vi "2.4b.vi"() -> ()   [LabVIEW 2020]
panel:
  out "output array 2":string[](array[string])
  in  "Array":string[][](array[string])
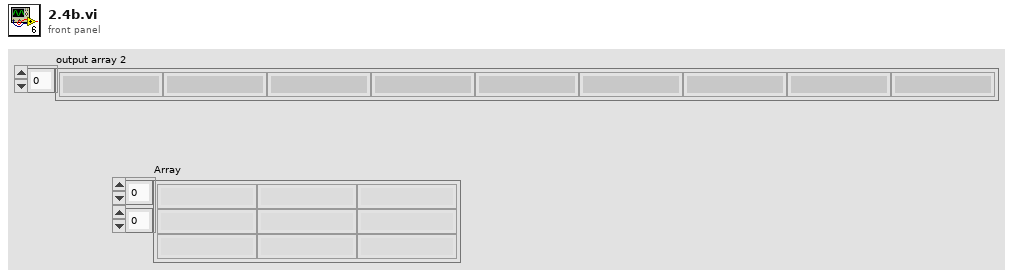
[diagram p1: front panel]
types:
  T1 = enum16{"open", "replace", "create", "open or create", "replace or create", "replace or create with confirmation"}
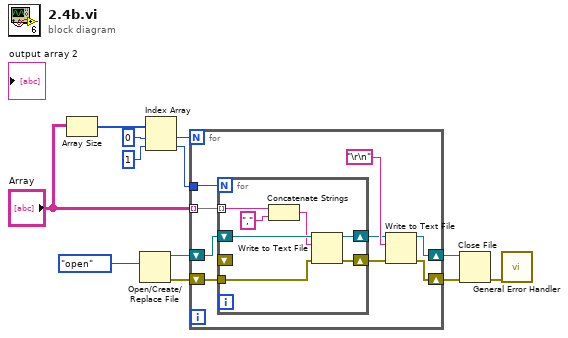
[diagram p0: block diagram]
diagram:
  n1 = Array Size(array="Array") -> (size(s)=w6:i32[])
  n2 = Open/Create/Replace File(operation (0:open)=T1."open") -> (refnum out=w11:refnum<file>, error out=w10:errorcluster)  [unwired: 5 in, 1 out]
  n3 = Index Array(array=w6, index #1=0 ("index"), index #2=1 ("index")) -> (element #1=w2:i32, element #2=w3:i32)
  n4 = for {
    N: w2 -> [_]
    shift-right: [w21] -> w9
    shift-left: w11 -> [w18]
    shift-right: [w20] -> w8
    shift-left: w10 -> [w17]
    tunnel: w3 -> [w19]
    tunnel: "Array" -> [w16] mode=indexing
    n5 = for {
      N: w19 -> [_]
      tunnel: w17 -> [w27]
      shift-right: [w26] -> w14
      shift-left: w18 -> [w28]
      tunnel: w16 -> [w23] mode=indexing
      shift-right: [w25] -> w13
      shift-left: _ -> [_]
      n6 = Concatenate Strings(w23, "," ("string")) -> (w22:string)
      n7 = Write to Text File(file (use dialog)=w28, text=w22, error in=w27) -> (refnum out=w26:refnum<file>, error out=w25:errorcluster)  [unwired: 1 in, 1 out]
    }
    n8 = Write to Text File(file (use dialog)=w14, text="\r\n", error in=w13) -> (refnum out=w21:refnum<file>, error out=w20:errorcluster)  [unwired: 1 in, 1 out]
  }
  n9 = Close File(refnum=w9, error in=w8) -> (error out=w7:errorcluster)  [unwired: 1 out]
  n10 = call <vilib>:"General Error Handler.vi"("error in (no error)"=w7) -> ()  [unwired: 10 in, 5 out]
